vi "InitDev.vi"(1 "SAVE?":bool, 2 "IP地址":string="192.168.1.16", 3 "SampleRate":T2(ring)=enum."105.468", 4 "SavePath":path) -> (0 "输出簇":T1)   [LabVIEW 2012]
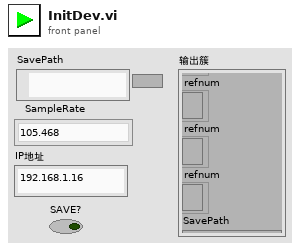
[diagram p1: front panel]
types:
  T1 = cluster{"refnum":refnum<file>, "refnum":refnum<file>, "refnum":refnum<file>, "refnum":refnum<file>, "refnum":refnum<file>, "SavePath":path, "SAVE?":bool, "connection ID":refnum<k5>}
  T2 = enum16{"", "105.468", "52.734", "35.156", "26.367", "21.094", "17.578", "15.067", "13.184", "11.719", "10.545"}
  T3 = enum16{"open", "replace", "create", "open or create", "replace or create", "replace or create with confirmation"}
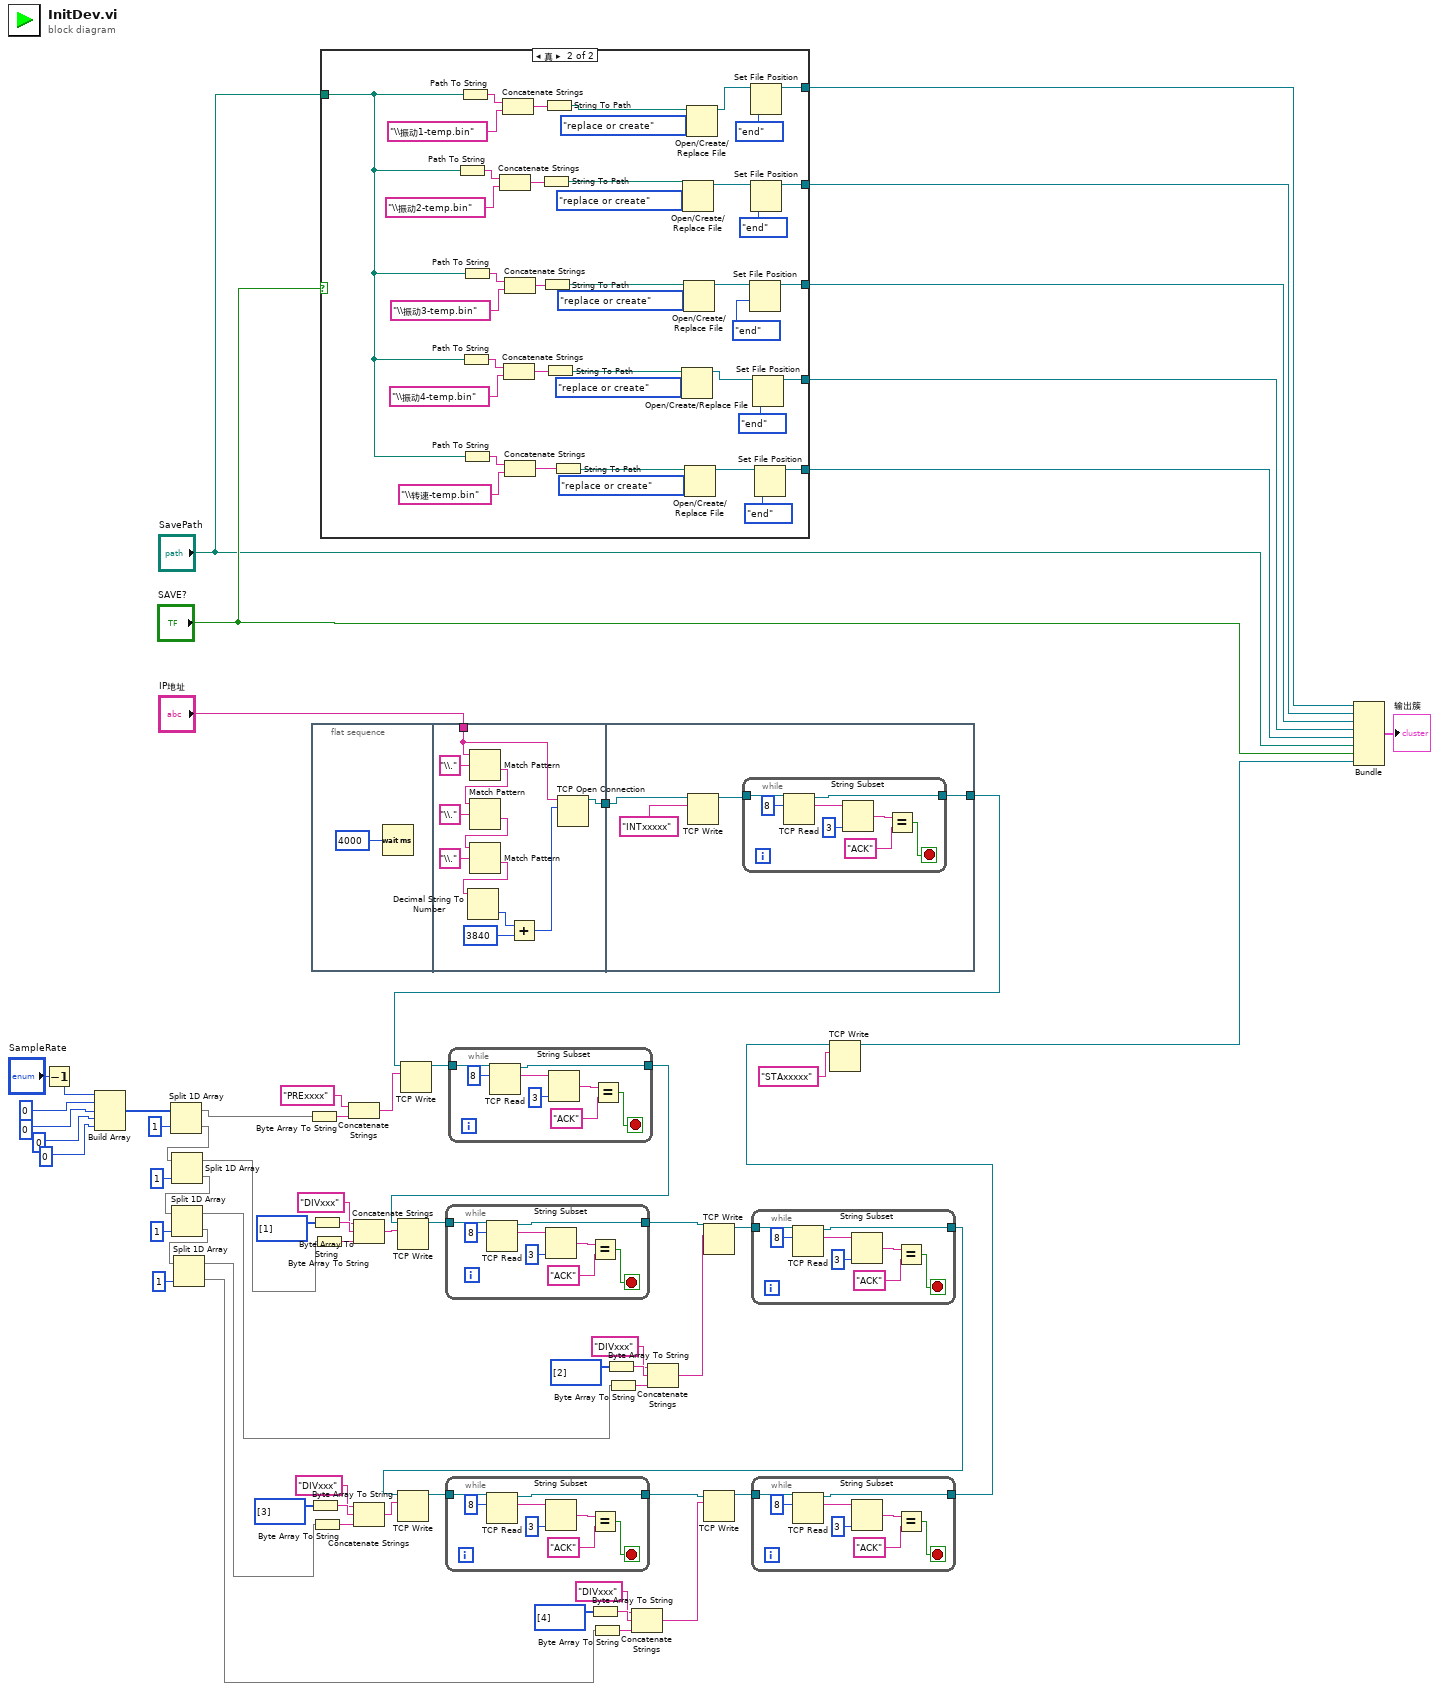
[diagram p0: block diagram]
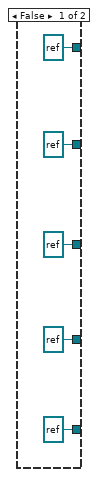
[diagram p2: hidden frame]
diagram:
  n1 = Decrement(x="SampleRate") -> (x-1=w9:T2)
  n2 = Build Array(w9, u8 0 ("元素"), u8 0 ("元素"), u8 0 ("元素"), u8 0 ("元素")) -> (w64:u16[])
  n3 = Split 1D Array(array=w64, index=1 ("索引")) -> (first subarray=w45:u16[], second subarray=w41:u16[])
  n4 = Split 1D Array(array=w41, index=1 ("索引")) -> (first subarray=w21:u16[], second subarray=w40:u16[])
  n5 = Split 1D Array(array=w40, index=1 ("索引")) -> (first subarray=w20:u16[], second subarray=w39:u16[])
  n6 = Split 1D Array(array=w39, index=1 ("索引")) -> (first subarray=w19:u16[], second subarray=w18:u16[])
  n7 = Byte Array To String(unsigned byte array=w45) -> (string=w49:string)
  n8 = Byte Array To String(unsigned byte array=u8[] [3] ("无符号字节数组")) -> (string=w27:string)
  n9 = flat-sequence {
    tunnel: [w77] -> w65
    tunnel: "IP地址" -> [w68]
    tunnel: w65 -> [w80]
    tunnel: [w78] -> w12
    frame #0 {
      n10 = Wait (ms)(milliseconds to wait=u32 4000 ("毫秒倍数")) -> ()  [unwired: 1 out]
    }
    frame #1 {
      n11 = Match Pattern(string=w68, regular expression="\\." ("正则表达式")) -> (after substring=w72:string)  [unwired: 1 in, 3 out]
      n12 = Match Pattern(string=w72, regular expression="\\." ("正则表达式")) -> (after substring=w73:string)  [unwired: 1 in, 3 out]
      n13 = Match Pattern(string=w73, regular expression="\\." ("正则表达式")) -> (after substring=w74:string)  [unwired: 1 in, 3 out]
      n14 = Decimal String To Number(string=w74) -> (number=w75:i32)  [unwired: 2 in, 1 out]
      n15 = Add(x=w75, y=3840) -> (x+y=w67:i32)
      n16 = TCP Open Connection(address=w68, remote port or service name=w67) -> (connection ID=w77:refnum<k5>)  [unwired: 3 in, 1 out]
    }
    frame #2 {
      n17 = TCP Write(connection ID=w80, data in="INTxxxxx" ("数据输入")) -> (connection ID out=w79:refnum<k5>)  [unwired: 2 in, 2 out]
      n18 = while {
        tunnel: w79 -> [w89]
        tunnel: [w83] -> w78
        stop <- w84 stop-if-true
        n19 = TCP Read(connection ID=w89, bytes to read=8 ("读取的字节")) -> (connection ID out=w83:refnum<k5>, data out=w87:string)  [unwired: 3 in, 1 out]
        n20 = String Subset(string=w87, length (rest)=3 ("偏移量(0)")) -> (substring=w86:string)  [unwired: 1 in]
        n21 = Equal?(x=w86, y="ACK") -> (x = y?=w84:bool)
      }
    }
  }
  n22 = Byte Array To String(unsigned byte array=u8[] [1] ("无符号字节数组")) -> (string=w35:string)
  n23 = Byte Array To String(unsigned byte array=w19) -> (string=w29:string)
  n24 = Byte Array To String(unsigned byte array=w21) -> (string=w38:string)
  n25 = case shown="真" "SAVE?" {
    tunnel: [refnum<file> refnum ("refnum") w115] -> w8
    tunnel: [refnum<file> refnum ("refnum") w114] -> w7
    tunnel: [refnum<file> refnum ("refnum") w113] -> w6
    tunnel: [refnum<file> refnum ("refnum") w112] -> w5
    tunnel: [refnum<file> refnum ("refnum") w111] -> w4
    tunnel: "SavePath" -> [_ w95]
    frame False {
    }
    frame True {
      n26 = Path To String(path=w95) -> (string=w109:string)
      n27 = Path To String(path=w95) -> (string=w110:string)
      n28 = Path To String(path=w95) -> (string=w107:string)
      n29 = Path To String(path=w95) -> (string=w108:string)
      n30 = Path To String(path=w95) -> (string=w106:string)
      n31 = Concatenate Strings(w109, "\\振动2-temp.bin" ("字符串")) -> (w99:string)
      n32 = Concatenate Strings(w110, "\\振动1-temp.bin" ("字符串")) -> (w100:string)
      n33 = Concatenate Strings(w107, "\\振动4-temp.bin" ("字符串")) -> (w97:string)
      n34 = Concatenate Strings(w108, "\\振动3-temp.bin" ("字符串")) -> (w98:string)
      n35 = Concatenate Strings(w106, "\\转速-temp.bin" ("字符串")) -> (w96:string)
      n36 = String To Path(string=w99) -> (path=w124:path)
      n37 = String To Path(string=w98) -> (path=w123:path)
      n38 = String To Path(string=w100) -> (path=w125:path)
      n39 = String To Path(string=w97) -> (path=w122:path)
      n40 = String To Path(string=w96) -> (path=w121:path)
      n41 = Open/Create/Replace File(file path (use dialog)=w122, operation (0:open)=T3."replace or create" ("操作(0:open)")) -> (refnum out=w132:refnum<file>)  [unwired: 4 in, 2 out]
      n42 = Open/Create/Replace File(file path (use dialog)=w124, operation (0:open)=T3."replace or create" ("操作(0:open)")) -> (refnum out=w134:refnum<file>)  [unwired: 4 in, 2 out]
      n43 = Open/Create/Replace File(file path (use dialog)=w123, operation (0:open)=T3."replace or create" ("操作(0:open)")) -> (refnum out=w133:refnum<file>)  [unwired: 4 in, 2 out]
      n44 = Open/Create/Replace File(file path (use dialog)=w121, operation (0:open)=T3."replace or create" ("操作(0:open)")) -> (refnum out=w131:refnum<file>)  [unwired: 4 in, 2 out]
      n45 = Open/Create/Replace File(file path (use dialog)=w125, operation (0:open)=T3."replace or create" ("操作(0:open)")) -> (refnum out=w135:refnum<file>)  [unwired: 4 in, 2 out]
      n46 = Set File Position(refnum=w133, from (0:start)=enum16{"start", "end", "current"}."end" ("自（0:起始）")) -> (refnum out=w113:refnum<file>)  [unwired: 2 in, 1 out]
      n47 = Set File Position(refnum=w135, from (0:start)=enum16{"start", "end", "current"}."end" ("自（0:起始）")) -> (refnum out=w115:refnum<file>)  [unwired: 2 in, 1 out]
      n48 = Set File Position(refnum=w134, from (0:start)=enum16{"start", "end", "current"}."end" ("自（0:起始）")) -> (refnum out=w114:refnum<file>)  [unwired: 2 in, 1 out]
      n49 = Set File Position(refnum=w132, from (0:start)=enum16{"start", "end", "current"}."end" ("自（0:起始）")) -> (refnum out=w112:refnum<file>)  [unwired: 2 in, 1 out]
      n50 = Set File Position(refnum=w131, from (0:start)=enum16{"start", "end", "current"}."end" ("自（0:起始）")) -> (refnum out=w111:refnum<file>)  [unwired: 2 in, 1 out]
    }
  }
  n51 = Concatenate Strings("PRExxxx" ("数据输入"), w49) -> (w47:string)
  n52 = Concatenate Strings("DIVxxx" ("数据输入"), w35, w38) -> (w37:string)
  n53 = Concatenate Strings("DIVxxx" ("数据输入"), w27, w29) -> (w13:string)
  n54 = TCP Write(connection ID=w12, data in=w47) -> (connection ID out=w58:refnum<k5>)  [unwired: 2 in, 2 out]
  n55 = while {
    tunnel: w58 -> [w143]
    tunnel: [w137] -> w53
    stop <- w138 stop-if-true
    n56 = TCP Read(connection ID=w143, bytes to read=8 ("读取的字节")) -> (connection ID out=w137:refnum<k5>, data out=w141:string)  [unwired: 3 in, 1 out]
    n57 = String Subset(string=w141, length (rest)=3 ("偏移量(0)")) -> (substring=w140:string)  [unwired: 1 in]
    n58 = Equal?(x=w140, y="ACK") -> (x = y?=w138:bool)
  }
  n59 = TCP Write(connection ID=w53, data in=w37) -> (connection ID out=w57:refnum<k5>)  [unwired: 2 in, 2 out]
  n60 = while {
    tunnel: w57 -> [w151]
    tunnel: [w145] -> w52
    stop <- w146 stop-if-true
    n61 = TCP Read(connection ID=w151, bytes to read=8 ("读取的字节")) -> (connection ID out=w145:refnum<k5>, data out=w149:string)  [unwired: 3 in, 1 out]
    n62 = String Subset(string=w149, length (rest)=3 ("偏移量(0)")) -> (substring=w148:string)  [unwired: 1 in]
    n63 = Equal?(x=w148, y="ACK") -> (x = y?=w146:bool)
  }
  n64 = Byte Array To String(unsigned byte array=u8[] [4] ("无符号字节数组")) -> (string=w23:string)
  n65 = Byte Array To String(unsigned byte array=w18) -> (string=w25:string)
  n66 = Byte Array To String(unsigned byte array=u8[] [2] ("无符号字节数组")) -> (string=w31:string)
  n67 = Byte Array To String(unsigned byte array=w20) -> (string=w33:string)
  n68 = Concatenate Strings("DIVxxx" ("数据输入"), w23, w25) -> (w16:string)
  n69 = Concatenate Strings("DIVxxx" ("数据输入"), w31, w33) -> (w17:string)
  n70 = TCP Write(connection ID=w52, data in=w17) -> (connection ID out=w56:refnum<k5>)  [unwired: 2 in, 2 out]
  n71 = while {
    tunnel: w56 -> [w159]
    tunnel: [w153] -> w51
    stop <- w154 stop-if-true
    n72 = TCP Read(connection ID=w159, bytes to read=8 ("读取的字节")) -> (connection ID out=w153:refnum<k5>, data out=w157:string)  [unwired: 3 in, 1 out]
    n73 = String Subset(string=w157, length (rest)=3 ("偏移量(0)")) -> (substring=w156:string)  [unwired: 1 in]
    n74 = Equal?(x=w156, y="ACK") -> (x = y?=w154:bool)
  }
  n75 = TCP Write(connection ID=w51, data in=w13) -> (connection ID out=w55:refnum<k5>)  [unwired: 2 in, 2 out]
  n76 = while {
    tunnel: w55 -> [w167]
    tunnel: [w161] -> w50
    stop <- w162 stop-if-true
    n77 = TCP Read(connection ID=w167, bytes to read=8 ("读取的字节")) -> (connection ID out=w161:refnum<k5>, data out=w165:string)  [unwired: 3 in, 1 out]
    n78 = String Subset(string=w165, length (rest)=3 ("偏移量(0)")) -> (substring=w164:string)  [unwired: 1 in]
    n79 = Equal?(x=w164, y="ACK") -> (x = y?=w162:bool)
  }
  n80 = TCP Write(connection ID=w50, data in=w16) -> (connection ID out=w54:refnum<k5>)  [unwired: 2 in, 2 out]
  n81 = while {
    tunnel: w54 -> [w175]
    tunnel: [w169] -> w15
    stop <- w170 stop-if-true
    n82 = TCP Read(connection ID=w175, bytes to read=8 ("读取的字节")) -> (connection ID out=w169:refnum<k5>, data out=w173:string)  [unwired: 3 in, 1 out]
    n83 = String Subset(string=w173, length (rest)=3 ("偏移量(0)")) -> (substring=w172:string)  [unwired: 1 in]
    n84 = Equal?(x=w172, y="ACK") -> (x = y?=w170:bool)
  }
  n85 = TCP Write(connection ID=w15, data in="STAxxxxx" ("数据输入")) -> (connection ID out=w11:refnum<k5>)  [unwired: 2 in, 2 out]
  n86 = Bundle("refnum"=w8, "refnum"=w7, "refnum"=w6, "refnum"=w5, "refnum"=w4, "SavePath"="SavePath", "SAVE?"="SAVE?", "connection ID"=w11) -> (→"输出簇":T1)  [unwired: 1 in]
